vi "PH_Image_Common.CalcPixelsum.vi"(0 "Image":T1, 5 "error in (no error)":errorcluster) -> (14 "Pixel Sum":sgl, 19 "error out":errorcluster)   [LabVIEW 2014, in "PH_Image_Common.lvlib"]
doc: "This VI calculates the sum by multiplying the number of pixels with the mean value over all pixels."
uses:
  <vilib>/vision/Image Controls.llb/IMAQ Image.ctl
  PH_Image_Common.lvlib
  <vilib>/vision/NI_Vision_Development_Module.lvlib
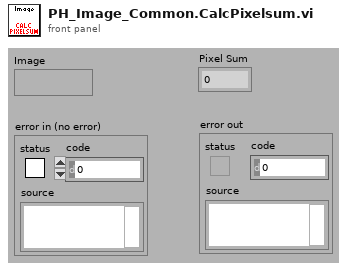
[diagram p1: front panel]
types:
  T1 = typedef "IMAQ Image.ctl" = refnum<image>
  T2 = cluster{"histogram":u32[], "Minimal Value":sgl, "Maximal Value":sgl, "Starting Value":sgl, "Interval Width":sgl, "Mean Value":sgl, "Standard  Variation":sgl, "Area (pixels)":i32}
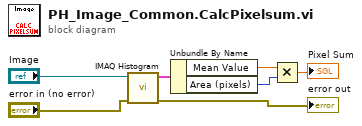
[diagram p0: block diagram]
diagram:
  n1 = call "IMAQ Histogram"("error in (no error)"="error in (no error)", "Image"="Image") -> ("error out"=→"error out":errorcluster, "Histogram Report"=w4:T2)  [unwired: 8 in]
  n2 = Unbundle By Name(w4) -> ("Mean Value"=w5:sgl, "Area (pixels)"=w6:i32)
  n3 = Multiply(x=w5, y=w6) -> (x*y=→"Pixel Sum":sgl)
